vi "TTOSEC.VI"(5 "String":string) -> (0 "Total Hours from Midnight":dbl format="%.4f", 1 "Total Minutes from Midnight":dbl format="%.4f", 2 "Total Seconds from Midnight":dbl format="%.4f", 4 "Array":string[](array[string]))   [LabVIEW 2014]
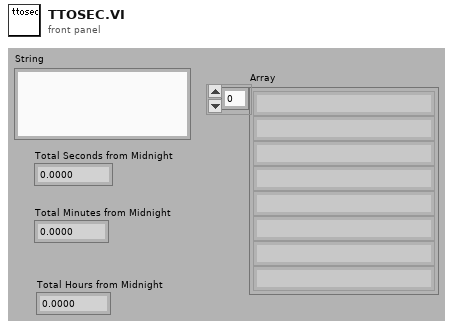
[diagram p1: front panel]
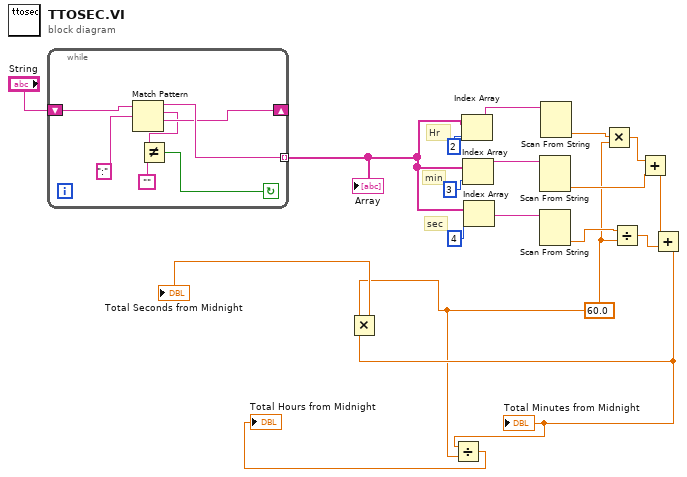
[diagram p0: block diagram]
diagram:
  w2 = 60.0
  # "sec"
  # "min"
  # "Hr"
  n1 = while {
    shift-right: [w21] -> _
    shift-left: "String" -> [w25]
    tunnel: [w23] -> w14 mode=indexing
    stop <- w19 continue-if-true
    n2 = Match Pattern(string=w25, regular expression=":") -> (before substring=w23:string, match substring=w20:string, after substring=w21:string)  [unwired: 1 in, 1 out]
    n3 = Not Equal?(x=w20, y="") -> (x != y?=w19:bool)
  }
  "Array" <- w14
  n4 = Index Array(array=w14, index=2) -> (element=w13:string)
  n5 = Index Array(array=w14, index=3) -> (element=w12:string)
  n6 = Index Array(array=w14, index=4) -> (element=w11:string)
  n7 = Scan From String(input string=w12) -> (output 1=w7:dbl)  [unwired: 4 in, 3 out]
  n8 = Scan From String(input string=w11) -> (output 1=w9:dbl)  [unwired: 4 in, 3 out]
  n9 = Scan From String(input string=w13) -> (output 1=w10:dbl)  [unwired: 4 in, 3 out]
  n10 = Multiply(x=w10, y=w2) -> (x*y=w8:dbl)
  n11 = Divide(x=w9, y=w2) -> (x/y=w5:dbl)
  n12 = Add(x=w8, y=w7) -> (x+y=w6:dbl)
  n13 = Add(x=w6, y=w5) -> (x+y=w3:dbl)
  "Total Minutes from Midnight" <- w3
  n14 = Multiply(x=w2, y=w3) -> (x*y=→"Total Seconds from Midnight":dbl)
  n15 = Divide(x=w3, y=w2) -> (x/y=→"Total Hours from Midnight":dbl)
